vi "polariser setup.vi"() -> ()   [LabVIEW 2014]
uses:
  <vilib>/Analysis/NI_AALBase.lvlib
panel:
  in  "Temp":sgl=30.0 min=10 max=50
  in  "Lcvr1 Voltage":dbl
  out "max beam":dbl[](array[numeric])
  out "min beam":dbl[](array[numeric])
  out "Equal Intensity ?":bool
  out "Y - centroid":dbl[](array[numeric])
  out "X - centroid":dbl[](array[numeric])
  in  "Exposure in msec":u32
  in  "OpenStructureIn":T1={"Size"=88, "InterfaceType"=1, "Camera Number"=0, "CameraNumAtInterface"=0, "OpenFlags"=[], "OpenDWFlags"=[], "OpenPtrs"=[]} {"InterfaceType" items=["IEEE1394/FireWire", "IEEE1394/FireWire", "Matrox Helios CameraLink", "SiliconSoftware MicroEnableIII CL", "National Instruments CameraLink", "Gigabit Ethernet", "USB", "SiliconSoftware MicroEnable IV CL", "Reserved", "Reserved", "Generic CameraLink with CLSER.DLL"]}
  in  "Start calibration":bool
  in  "OK":bool
  out "Horizontal ?":bool
  out "Intensity Graph":u16[][](graph)
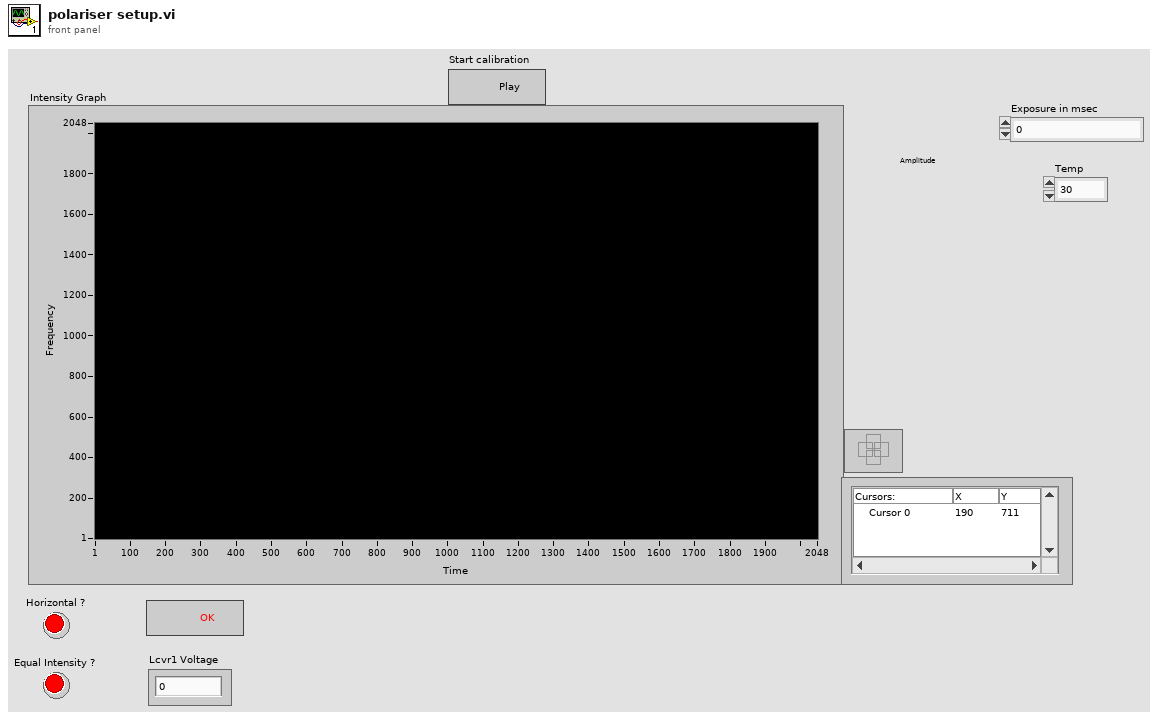
[diagram p1: front panel]
types:
  T1 = cluster{"Size":u16, "InterfaceType":u16, "Camera Number":u16, "CameraNumAtInterface":u16, "OpenFlags":u16[], "OpenDWFlags":u32[], "OpenPtrs":u32[]}
  T2 = cluster{"Device Handle":u32, "Pipe 0 Handle":u32, "Pipe 1 Handle":u32}[]
  T3 = cluster{"Device Handle":u32, "Pipe 0 Handle":u32, "Pipe 1 Handle":u32}
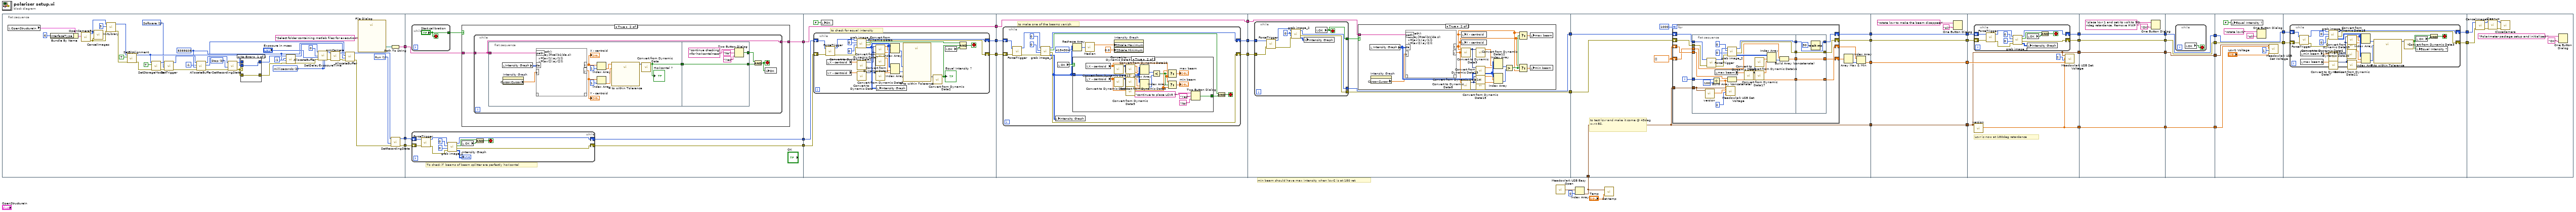
[diagram p0: block diagram]
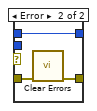
[diagram p2: hidden frame]
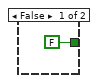
[diagram p4: hidden frame]
diagram:
  # "min beam should have max intensity when lcvr2 is at 180 ret"
  n1 = flat-sequence {
    tunnel: [w55] -> w42
    tunnel: [w54] -> w41
    tunnel: [w50] -> w4
    tunnel: w42 -> [w98]
    tunnel: w41 -> [w97]
    tunnel: [w96] -> w40
    tunnel: [w95] -> w39
    tunnel: w4 -> [w94]
    tunnel: [w93] -> w1
    tunnel: w40 -> [w142]
    tunnel: w39 -> [w141]
    tunnel: [w140] -> w38
    tunnel: [w139] -> w37
    tunnel: [w138] -> w2
    tunnel: w1 -> [w138]
    tunnel: w38 -> [w171]
    tunnel: w37 -> [w170]
    tunnel: [w169] -> w8
    tunnel: [w168] -> w6
    tunnel: [w167] -> w3
    tunnel: w2 -> [w167]
    tunnel: w8 -> [w213]
    tunnel: [w212] -> w7
    tunnel: w6 -> [w211]
    tunnel: [w210] -> w5
    tunnel: w3 -> [w208]
    tunnel: w7 -> [w248]
    tunnel: w5 -> [w247]
    tunnel: [w242] -> w36
    tunnel: [w239] -> w34
    tunnel: [w241] -> w31
    tunnel: [w240] -> w29
    tunnel: w10 -> [w239]
    tunnel: w36 -> [w298]
    tunnel: [w298] -> w35
    tunnel: w34 -> [w297]
    tunnel: [w297] -> w33
    tunnel: [w294] -> w32
    tunnel: w31 -> [w294]
    tunnel: [w293] -> w30
    tunnel: w29 -> [w293]
    tunnel: w35 -> [w306]
    tunnel: w33 -> [w302]
    tunnel: w32 -> [w304]
    tunnel: w30 -> [w303]
    tunnel: [w302] -> w28
    tunnel: [w301] -> w27
    tunnel: [w300] -> w19
    tunnel: [w299] -> w15
    tunnel: [w322] -> w26
    tunnel: w28 -> [w322]
    tunnel: [w321] -> w24
    tunnel: w27 -> [w321]
    tunnel: [w320] -> w20
    tunnel: w19 -> [w320]
    tunnel: [w319] -> w16
    tunnel: w15 -> [w319]
    tunnel: w26 -> [w328]
    tunnel: [w328] -> w25
    tunnel: w24 -> [w327]
    tunnel: [w327] -> w23
    tunnel: [w326] -> w21
    tunnel: w20 -> [w326]
    tunnel: [w325] -> w17
    tunnel: w16 -> [w325]
    tunnel: w25 -> [w338]
    tunnel: w23 -> [w337]
    tunnel: [w332] -> w22
    tunnel: w21 -> [w332]
    tunnel: [w331] -> w18
    tunnel: w17 -> [w331]
    tunnel: w22 -> [w342]
    tunnel: w18 -> [w341]
    tunnel: [w340] -> w14
    tunnel: [w339] -> w13
    tunnel: w14 -> [w371]
    tunnel: w13 -> [w370]
    frame #0 {
      w56 = u16 1 items=["Stop", "Run"] ("RecordingState")
      w60 = u16 1 items=["Auto", "Software", "External sequence start ", "External exposure control"] ("TriggerMode")
      w69 = u16 2 items=["nanoseconds", "microseconds", "milliseconds"] ("ExposureTimeBase")
      w45 = u32 8388608 ("Size")
      w79 = u16 0 items=["Stop", "Run"] ("RecordingState")
      n2 = local read "OpenStructureIn"() -> (w87:T1)
      n3 = Bundle By Name(cluster=w87, "InterfaceType"=u16 6) -> (w85:T1)
      n4 = call <userlib>:"OpenCameraEx.vi"("OpenStructureIn"=w85) -> ("error out"=w83:errorcluster, "hout"=w84:u64)  [unwired: 3 in, 2 out]
      n5 = call <userlib>:"CancelImages.vi"("error in (no error)"=w83, "ph"=w84) -> ()  [unwired: 1 in, 3 out]
      n6 = call <userlib>:"InitLibrary.vi"("error in (no error)"=w83, "InterfaceType"=u32 3, "ph"=w84) -> ("error out"=w80:errorcluster, "hout"=w81:u64)  [unwired: 7 in]
      n7 = call <userlib>:"SetBitAlignment.vi"("error in (no error)"=w80, "BitAlignent"=TRUE, "ph"=w81) -> ("error out"=w59:errorcluster, "hout"=w64:u64)  [unwired: 2 in, 1 out]
      n8 = call <userlib>:"SetStorageMode.vi"("error in (no error)"=w59, "StorageMode"=TRUE, "ph"=w64) -> ("error out"=w61:errorcluster, "hout"=w62:u64)  [unwired: 2 in, 1 out]
      n9 = call <userlib>:"SetTrigger.vi"("error in (no error)"=w61, "TriggerMode"=w60, "ph"=w62) -> ("error out"=w47:errorcluster, "hout"=w49:u64)  [unwired: 2 in, 1 out]
      n10 = call <userlib>:"AllocateBuffer.vi"("error in (no error)"=w47, "Size"=w45, "BufNr"=i16 -1, "ph"=w49) -> ("error out"=w46:errorcluster, "BufNrOut"=w43:i16, "hout"=w48:u64)  [unwired: 2 in, 3 out]
      n11 = call <userlib>:"SetRecordingState.vi"("ErrorIn"=w46, "RecordingState"=w79, "ph"=w48) -> ("ErrorOut"=w77:errorcluster, "hout"=w78:u64)  [unwired: 2 in, 1 out]
      n12 = case shown="No Error" w77 {
        tunnel: [w89 w91] -> w75
        tunnel: w77 -> [w89 w92]
        tunnel: w78 -> [w88 _]
        tunnel: [w88 w90] -> w76
        tunnel: w64 -> [_ w90]
        frame No Error {
        }
        frame Error {
          n13 = call <vilib>:"Clear Errors.vi"("error in (no error)"=w92) -> ("error out"=w91:errorcluster)  [unwired: 5 in, 1 out]
        }
      }
      n14 = call <userlib>:"AllocateBuffer.vi"("error in (no error)"=w75, "Size"=w45, "BufNr"=i16 -1, "ph"=w76) -> ("error out"=w72:errorcluster, "hout"=w73:u64)  [unwired: 2 in, 4 out]
      n15 = call <userlib>:"SetDelayExposureTime.vi"("ph"=w73, "Delay"=u32 0, "Exposure"="Exposure in msec", "error in (no error)"=w72, "DelayTimeBase"=w69, "ExposureTimeBase"=w69) -> ("hout"=w68:u64, "error out"=w67:errorcluster)  [unwired: 7 in, 1 out]
      n16 = call <userlib>:"ArmCamera.vi"("error in (no error)"=w67, "ph"=w68) -> ("error out"=w65:errorcluster, "hout"=w66:u64)  [unwired: 2 out]
      n17 = call <userlib>:"AllocateBuffer.vi"("error in (no error)"=w65, "Size"=w45, "BufNr"=w43, "ph"=w66) -> ("error out"=w57:errorcluster, "hout"=w58:u64)  [unwired: 2 in, 4 out]
      n18 = call "File Dialog"("prompt"="Select folder containing matlab files for execution") -> ("selected path"=w51:path)  [unwired: 11 in, 3 out]
      n19 = Path To String(path=w51) -> (string=w50:string)
      n20 = call <userlib>:"SetRecordingState.vi"("ErrorIn"=w57, "RecordingState"=w56, "ph"=w58) -> ("ErrorOut"=w54:errorcluster, "hout"=w55:u64)  [unwired: 2 in, 1 out]
    }
    frame #1 {
      # "To check if  beams of beam splitter are perfectly horizontal"
      n21 = while {
        tunnel: ["Start calibration"] -> w99
        stop <- "Start calibration" stop-if-true
      }
      n22 = while {
        shift-right: [w106] -> w96
        shift-left: w98 -> [w112]
        shift-right: [w105] -> w95
        shift-left: w97 -> [w111]
        stop <- w101 stop-if-true
        n23 = call <userlib>:"ForceTrigger.vi"("ph"=w112, "error in (no error)"=w111) -> ("hout"=w110:u64, "error out"=w109:errorcluster)  [unwired: 1 in, 2 out]
        n24 = call "grab image_2.vi"("ErrorIn"=w109, "Image number"=u32 0, "BuffNr"=i16 0, "ph"=w110) -> ("output image"=→"Intensity Graph":u16[][], "error out"=w105:errorcluster, "Buffer_Ready"=w102:bool, "hout"=w106:u64)  [unwired: 4 in]
        n25 = local read "OK"() -> (w103:bool)
        n26 = And(x=w102, y=w103) -> (x .and. y?=w101:bool)
      }
      n27 = case shown="True" w99 {
        tunnel: w94 -> [w113 w115]
        tunnel: [w113 w114] -> w93
        frame False {
        }
        frame True {
          n28 = while {
            tunnel: w115 -> [w120]
            tunnel: [w120] -> w114
            stop <- w116 stop-if-true
            n29 = flat-sequence {
              tunnel: w120 -> [w122]
              tunnel: [w121] -> w117
              tunnel: [w133] -> w119
              tunnel: [w132] -> w118
              tunnel: w117 -> [w132]
              frame #0 {
                n30 = local read "Intensity Graph"() -> (w126:u16[][])
                n31 = property on="Intensity Graph" class="IntGraph (strict)"() -> ("Cursor.Cursor X"=w125:dbl)  [unwired: 2 in, 2 out]
                n32 = script code="cd(path);\n[ax,ay]=calib1(da,s);\nx=[ax(1),ay(1)];\ny=[ax(2),ay(2)];"("path"=w122, "da"=w126, "s"=w125) -> ("x"=w124:dbl[], "y"=w123:dbl[])  [unwired: 1 in, 1 out]
                "X - centroid" <- w124
                "Y - centroid" <- w123
                n33 = Index Array(array=w124, index=1) -> (element=w129:dbl)
                n34 = Index Array(array=w123, index=1) -> (element=w128:dbl)
                n35 = call "= to within Tolerance"("Operand 2"=w128, "Operand 1"=w129) -> ("Result"=w127:dynamicdata)  [unwired: 8 in, 1 out]
                n36 = call "Convert from Dynamic Data"("Dynamic Data Type"=w127) -> ("Scalar"=w121:bool)  [unwired: 3 in]
                "Horizontal ?" <- w121
              }
              frame #1 {
                n37 = Two Button Dialog(message="continue checking\nfor horizontalness", 1:"Yes" ("F button name (\"Cancel\")"), 2:"No" ("T button name (\"OK\")")) -> (T button?=w133:bool)
              }
            }
            n38 = And(x=w119, y=w118) -> (x .and. y?=w116:bool)
            n39 = local write "OK"(w116) -> ()
          }
        }
      }
    }
    frame #2 {
      # "to check for equal intensity"
      n40 = while {
        shift-right: [w162] -> w140
        shift-left: w142 -> [w166]
        shift-right: [w161] -> w139
        shift-left: w141 -> [w165]
        stop <- w150 stop-if-true
        n41 = call <userlib>:"ForceTrigger.vi"("ph"=w166, "error in (no error)"=w165) -> ("hout"=w164:u64, "error out"=w163:errorcluster)  [unwired: 1 in, 2 out]
        n42 = local read "X - centroid"() -> (w155:dbl[])
        n43 = local read "Y - centroid"() -> (w156:dbl[])
        n44 = call "grab image_2.vi"("ErrorIn"=w163, "Image number"=u32 0, "BuffNr"=i16 0, "ph"=w164) -> ("output image"=w158:u16[][], "error out"=w161:errorcluster, "Buffer_Ready"=w149:bool, "hout"=w162:u64)  [unwired: 4 in]
        n45 = call "Convert to Dynamic Data2"("Array"=w155) -> ("Dynamic Data Type"=w145:dynamicdata)  [unwired: 3 in]
        n46 = call "Convert to Dynamic Data"("Array"=w156) -> ("Dynamic Data Type"=w148:dynamicdata)  [unwired: 3 in]
        n47 = call "Convert from Dynamic Data6"("Dynamic Data Type"=w145) -> ("Scalar"=w144:dbl)  [unwired: 3 in]
        n48 = call "Convert from Dynamic Data7"("Dynamic Data Type"=w145) -> ("Scalar"=w143:dbl)  [unwired: 3 in]
        n49 = call "Convert from Dynamic Data4"("Dynamic Data Type"=w148) -> ("Scalar"=w147:dbl)  [unwired: 3 in]
        n50 = call "Convert from Dynamic Data5"("Dynamic Data Type"=w148) -> ("Scalar"=w146:dbl)  [unwired: 3 in]
        n51 = local write "Intensity Graph"(w158) -> ()
        n52 = Index Array(array=w158, index (row)=w144, index (col)=w143) -> (element=w153:u16)
        n53 = Index Array(array=w158, index (row)=w147, index (col)=w146) -> (element=w154:u16)
        n54 = call "= to within Tolerance"("Operand 2"=w154, "Operand 1"=w153) -> ("Result"=w157:dynamicdata)  [unwired: 8 in, 1 out]
        n55 = call "Convert from Dynamic Data2"("Dynamic Data Type"=w157) -> ("Scalar"=w152:bool)  [unwired: 3 in]
        "Equal Intensity ?" <- w152
        n56 = local read "OK"() -> (w151:bool)
        n57 = Compound Arithmetic op=AND(w149, w152, w151) -> (w150:bool)
      }
      n58 = local write "OK"(FALSE ("OK")) -> ()
    }
    frame #3 {
      # "to make one of the beams vanish"
      n59 = while {
        shift-right: [w186] -> w169
        shift-left: w171 -> [w188]
        shift-right: [w183] -> w168
        shift-left: w170 -> [w185]
        stop <- w173 stop-if-true
        n60 = call <userlib>:"ForceTrigger.vi"("ph"=w188, "error in (no error)"=w185) -> ("hout"=w187:u64, "error out"=w184:errorcluster)  [unwired: 1 in, 2 out]
        n61 = call "grab image_2.vi"("ErrorIn"=w184, "Image number"=u32 0, "BuffNr"=i16 0, "ph"=w187) -> ("output image"=w172:u16[][], "error out"=w183:errorcluster, "Buffer_Ready"=w174:bool, "hout"=w186:u64)  [unwired: 4 in]
        n62 = local write "Intensity Graph"(w172) -> ()
        n63 = local read "OK"() -> (w176:bool)
        n64 = Reshape Array(w172, 4194304 ("dimension size")) -> (w180:u16[])
        n65 = case shown="True" w176 {
          tunnel: [FALSE w207] -> w175
          tunnel: w172 -> [_ w203]
          frame False {
          }
          frame True {
            n66 = local read "X - centroid"() -> (w199:dbl[])
            n67 = local read "Y - centroid"() -> (w198:dbl[])
            n68 = call "Convert to Dynamic Data3"("Array"=w199) -> ("Dynamic Data Type"=w192:dynamicdata)  [unwired: 3 in]
            n69 = call "Convert to Dynamic Data4"("Array"=w198) -> ("Dynamic Data Type"=w195:dynamicdata)  [unwired: 3 in]
            n70 = call "Convert from Dynamic Data10"("Dynamic Data Type"=w192) -> ("Scalar"=w191:dbl)  [unwired: 3 in]
            n71 = call "Convert from Dynamic Data11"("Dynamic Data Type"=w192) -> ("Scalar"=w190:dbl)  [unwired: 3 in]
            n72 = call "Convert from Dynamic Data8"("Dynamic Data Type"=w195) -> ("Scalar"=w194:dbl)  [unwired: 3 in]
            n73 = call "Convert from Dynamic Data9"("Dynamic Data Type"=w195) -> ("Scalar"=w193:dbl)  [unwired: 3 in]
            n74 = Index Array(array=w203, index (row)=w191, index (col)=w190) -> (element=w202:u16)
            n75 = Index Array(array=w203, index (row)=w194, index (col)=w193) -> (element=w201:u16)
            n76 = Less?(x=w202, y=w201) -> (x < y?=w197:bool)
            n77 = Select(t=w198, s=w197, f=w199) -> (s? t:f=→"max beam":dbl[])
            n78 = Select(t=w199, s=w197, f=w198) -> (s? t:f=→"min beam":dbl[])
            n79 = Two Button Dialog(message="continue to place LCVR ?", 1:"No" ("F button name (\"Cancel\")"), 2:"Yes" ("T button name (\"OK\")")) -> (T button?=w207:bool)
          }
        }
        n80 = call <vilib>:"Median.vi"("X"=w180) -> ("median"=w178:dbl)  [unwired: 1 out]
        n81 = property on="Intensity Graph" class="IntGraph (strict)"("ZScale.Maximum"=w178, "ZScale.Minimum"=0.0 ("Z Scale.Range:Minimum")) -> ()  [unwired: 2 in, 2 out]
        n82 = And(x=w174, y=w175) -> (x .and. y?=w173:bool)
      }
    }
    frame #4 {
      n83 = while {
        tunnel: w213 -> [w222]
        tunnel: w211 -> [w221]
        tunnel: [w217] -> w212
        tunnel: [w216] -> w210
        tunnel: [w215] -> w209
        stop <- w215 stop-if-true
        w218 = i16 0 ("BuffNr")
        n84 = call <userlib>:"ForceTrigger.vi"("ph"=w222, "error in (no error)"=w221) -> ("hout"=w220:u64, "error out"=w219:errorcluster)  [unwired: 1 in, 2 out]
        n85 = call "grab image_2.vi"("ErrorIn"=w219, "Image number"=w218, "BuffNr"=w218, "ph"=w220) -> ("output image"=w214:u16[][], "error out"=w216:errorcluster, "hout"=w217:u64)  [unwired: 4 in, 1 out]
        n86 = local write "Intensity Graph"(w214) -> ()
        n87 = local read "OK"() -> (w215:bool)
      }
      n88 = case shown="True" w209 {
        tunnel: w208 -> [_ w233]
        frame False {
        }
        frame True {
          n89 = local read "Intensity Graph"() -> (w232:u16[][])
          n90 = property on="Intensity Graph" class="IntGraph (strict)"() -> ("Cursor.Cursor X"=w229:dbl)  [unwired: 2 in, 2 out]
          n91 = script code="cd(path);\n[ax,ay]=calib1(da,s);\nx=[ax(1),ay(1)];\ny=[ax(2),ay(2)];"("path"=w233, "da"=w232, "s"=w229) -> ("x"=w231:dbl[], "y"=w230:dbl[])  [unwired: 1 in, 1 out]
          n92 = call "Convert to Dynamic Data9"("Array"=w231) -> ("Dynamic Data Type"=w228:dynamicdata)  [unwired: 3 in]
          n93 = call "Convert to Dynamic Data8"("Array"=w230) -> ("Dynamic Data Type"=w225:dynamicdata)  [unwired: 3 in]
          n94 = local write "X - centroid"(w231) -> ()
          n95 = local write "Y - centroid"(w230) -> ()
          n96 = call "Convert from Dynamic Data12"("Dynamic Data Type"=w228) -> ("Scalar"=w227:dbl)  [unwired: 3 in]
          n97 = call "Convert from Dynamic Data13"("Dynamic Data Type"=w228) -> ("Scalar"=w226:dbl)  [unwired: 3 in]
          n98 = call "Convert from Dynamic Data14"("Dynamic Data Type"=w225) -> ("Scalar"=w224:dbl)  [unwired: 3 in]
          n99 = call "Convert from Dynamic Data15"("Dynamic Data Type"=w225) -> ("Scalar"=w223:dbl)  [unwired: 3 in]
          n100 = Index Array(array=w232, index (row)=w227, index (col)=w226) -> (element=w238:u16)
          n101 = Index Array(array=w232, index (row)=w224, index (col)=w223) -> (element=w237:u16)
          n102 = Greater?(x=w238, y=w237) -> (0:w235:bool)
          n103 = Select(t=w231, s=w235, f=w230) -> (s? t:f=w236:dbl[])
          n104 = Select(t=w230, s=w235, f=w231) -> (s? t:f=w234:dbl[])
          n105 = local write "max beam"(w236) -> ()
          n106 = local write "min beam"(w234) -> ()
        }
      }
    }
    frame #5 {
      w246 = dbl[] []
      # "to test lcvr and make it come @ 45deg w.r.t BS."
      n107 = for {
        N: 1000 -> [_]
        tunnel: w239 -> [w263]
        shift-right: [w260] -> w244
        shift-left: w246 -> [w261]
        shift-right: [w258] -> w241
        shift-left: w248 -> [w259]
        shift-right: [w256] -> w240
        shift-left: w247 -> [w257]
        shift-right: [w255] -> w245
        shift-left: w246 -> [w254]
        i -> [w262]
        n108 = flat-sequence {
          tunnel: w263 -> [w286]
          tunnel: w262 -> [w284]
          tunnel: w261 -> [w281]
          tunnel: w259 -> [w275]
          tunnel: w257 -> [w273]
          tunnel: w254 -> [w267]
          tunnel: [w280] -> w253
          tunnel: [w274] -> w252
          tunnel: [w272] -> w251
          tunnel: [w268] -> w250
          tunnel: [w289] -> w255
          tunnel: [w290] -> w256
          tunnel: [w291] -> w258
          tunnel: [w292] -> w260
          tunnel: w253 -> [w292]
          tunnel: w252 -> [w291]
          tunnel: w251 -> [w290]
          tunnel: w250 -> [w289]
          frame #0 {
            n109 = call <userlib>:"version.vi"("USB Open Device Cluster"=w286) -> ("Version"=w287:dbl)  [unwired: 10 in]
            n110 = call <userlib>:"ForceTrigger.vi"("ph"=w275, "error in (no error)"=w273) -> ("hout"=w279:u64, "error out"=w278:errorcluster)  [unwired: 1 in, 2 out]
            n111 = Divide(x=w284, y=100) -> (x/y=w282:dbl)
            n112 = local read "max beam"() -> (w270:dbl[])
            n113 = call <userlib>:"Meadowlark USB Set Voltage.VI"("LC Voltage"=w282, "LC Channel"=2, "FW Version"=w287, "USB Open Device Cluster"=w286) -> ()  [unwired: 1 out]
            n114 = call "grab image_2.vi"("ErrorIn"=w278, "Image number"=u32 0, "BuffNr"=i16 0, "ph"=w279) -> ("output image"=w271:u16[][], "error out"=w272:errorcluster, "hout"=w274:u64)  [unwired: 4 in, 1 out]
            n115 = Build Array (concatenate)(w281, w282) -> (w280:dbl[])
            n116 = call "Convert to Dynamic Data5"("Array"=w270) -> ("Dynamic Data Type"=w266:dynamicdata)  [unwired: 3 in]
            n117 = call "Convert from Dynamic Data16"("Dynamic Data Type"=w266) -> ("Scalar"=w265:dbl)  [unwired: 3 in]
            n118 = call "Convert from Dynamic Data17"("Dynamic Data Type"=w266) -> ("Scalar"=w264:dbl)  [unwired: 3 in]
            n119 = Index Array(array=w271, index (row)=w265, index (col)=w264) -> (element=w269:u16)
            n120 = Build Array (concatenate)(w267, w269) -> (w268:dbl[])
          }
          frame #1 {
            n121 = Wait (ms)(milliseconds to wait=u32 30) -> ()  [unwired: 1 out]
          }
        }
      }
      n122 = Array Max & Min(array=w245) -> (min index (indices)=w243:i32)  [unwired: 3 out]
      n123 = Index Array(array=w244, index=w243) -> (element=w242:dbl)
    }
    frame #6 {
      n124 = One Button Dialog(message="rotate lcvr to make the beam disappear", button name ("OK")="ok") -> ()  [unwired: 1 out]
    }
    frame #7 {
      # "Lcvr is now at 180deg retardance"
      n125 = while {
        shift-right: [w314] -> w299
        shift-left: w303 -> [w315]
        shift-right: [w316] -> w300
        shift-left: w304 -> [w311]
        stop <- w307 stop-if-true
        n126 = call <userlib>:"ForceTrigger.vi"("ph"=w311, "error in (no error)"=w315) -> ("hout"=w318:u64, "error out"=w317:errorcluster)  [unwired: 1 in, 2 out]
        n127 = call "grab image_2.vi"("ErrorIn"=w317, "Image number"=u32 0, "BuffNr"=i16 0, "ph"=w318) -> ("output image"=w310:u16[][], "error out"=w314:errorcluster, "Buffer_Ready"=w309:bool, "hout"=w316:u64)  [unwired: 4 in]
        n128 = local read "OK"() -> (w308:bool)
        n129 = local write "Intensity Graph"(w310) -> ()
        n130 = And(x=w309, y=w308) -> (x .and. y?=w307:bool)
      }
      n131 = call <userlib>:"version.vi"("USB Open Device Cluster"=w302) -> ("Version"=w301:dbl)  [unwired: 10 in]
      n132 = call <userlib>:"Meadowlark USB Set Voltage.VI"("LC Voltage"=w306, "LC Channel"=2, "FW Version"=w301, "USB Open Device Cluster"=w302) -> ()  [unwired: 1 out]
    }
    frame #8 {
      n133 = One Button Dialog(message="place lcvr 1 and set its volt to 90\ndeg retardance. Remove HWP ", button name ("OK")="OK") -> ()  [unwired: 1 out]
    }
    frame #9 {
      n134 = while {
        stop <- w329 stop-if-true
        n135 = local read "OK"() -> (w329:bool)
      }
    }
    frame #10 {
      n136 = local write "Equal Intensity ?"(FALSE ("Equal Intensity ?")) -> ()
      n137 = One Button Dialog(message="rotate lcvr1", button name ("OK")="ok") -> ()  [unwired: 1 out]
      n138 = call <userlib>:"Meadowlark USB Set Voltage.VI"("LC Voltage"="Lcvr1 Voltage", "LC Channel"=1, "FW Version"=w337, "USB Open Device Cluster"=w338) -> ()  [unwired: 1 out]
    }
    frame #11 {
      n139 = while {
        shift-right: [w360] -> w340
        shift-left: w342 -> [w363]
        shift-right: [w358] -> w339
        shift-left: w341 -> [w362]
        stop <- w350 stop-if-true
        n140 = call <userlib>:"ForceTrigger.vi"("ph"=w363, "error in (no error)"=w362) -> ("hout"=w361:u64, "error out"=w359:errorcluster)  [unwired: 1 in, 2 out]
        n141 = local read "min beam"() -> (w365:dbl[])
        n142 = local read "max beam"() -> (w364:dbl[])
        n143 = call "grab image_2.vi"("ErrorIn"=w359, "Image number"=u32 0, "BuffNr"=i16 0, "ph"=w361) -> ("output image"=w355:u16[][], "error out"=w358:errorcluster, "hout"=w360:u64)  [unwired: 4 in, 1 out]
        n144 = call "Convert to Dynamic Data6"("Array"=w365) -> ("Dynamic Data Type"=w348:dynamicdata)  [unwired: 3 in]
        n145 = call "Convert to Dynamic Data7"("Array"=w364) -> ("Dynamic Data Type"=w345:dynamicdata)  [unwired: 3 in]
        n146 = call "Convert from Dynamic Data20"("Dynamic Data Type"=w345) -> ("Scalar"=w344:dbl)  [unwired: 3 in]
        n147 = call "Convert from Dynamic Data18"("Dynamic Data Type"=w348) -> ("Scalar"=w347:dbl)  [unwired: 3 in]
        n148 = call "Convert from Dynamic Data19"("Dynamic Data Type"=w348) -> ("Scalar"=w346:dbl)  [unwired: 3 in]
        n149 = call "Convert from Dynamic Data21"("Dynamic Data Type"=w345) -> ("Scalar"=w343:dbl)  [unwired: 3 in]
        n150 = Index Array(array=w355, index (row)=w347, index (col)=w346) -> (element=w354:u16)
        n151 = Index Array(array=w355, index (row)=w344, index (col)=w343) -> (element=w353:u16)
        n152 = call "= to within Tolerance"("Operand 2"=w353, "Operand 1"=w354) -> ("Result"=w351:dynamicdata)  [unwired: 8 in, 1 out]
        n153 = call "Convert from Dynamic Data3"("Dynamic Data Type"=w351) -> ("Scalar"=w349:bool)  [unwired: 3 in]
        n154 = local read "OK"() -> (w352:bool)
        n155 = local write "Equal Intensity ?"(w349) -> ()
        n156 = And(x=w349, y=w352) -> (x .and. y?=w350:bool)
      }
    }
    frame #12 {
      n157 = call <userlib>:"CancelImages.vi"("error in (no error)"=w370, "ph"=w371) -> ("error out"=w368:errorcluster, "hout"=w369:u64)  [unwired: 1 in, 1 out]
      n158 = call <userlib>:"Cleanup.vi"("error in (no error)"=w368, "ph"=w369) -> ("error out"=w366:errorcluster, "hout"=w367:u64)  [unwired: 8 in]
      n159 = call <userlib>:"CloseCamera.vi"("ErrorIn"=w366, "Handle in"=w367) -> ()  [unwired: 1 in, 3 out]
      n160 = One Button Dialog(message="Polarimeter package setup and initialised ", button name ("OK")="OK") -> ()  [unwired: 1 out]
    }
  }
  n161 = call <userlib>:"Meadowlark USB Easy Open.vi"() -> ("USB Device and Pipes Array"=w11:T2)  [unwired: 2 out]
  n162 = Index Array(array=w11, index=0) -> (element=w10:T3)
  n163 = call <userlib>:"Set temp.vi"("Temp"="Temp", "USB Open Device Cluster"=w10) -> ()  [unwired: 1 in]
